vi "Store File Header.vi"(0 "∆ Trigger":dbl format="%.2f", 1 "Trigger Column":u32, 2 "Comments":string="This data's for you!\nType Command\u0011-H to get a help window for the various controls.", 4 "Offsets":dbl[](array[numeric]) format="%_6e", 6 "Scale Factors":dbl[](array[numeric]) format="%_6e", 7 "Output File Name":string, 10 "User Name":string="Conan The Scientist", 11 "File Ref Num In":refnum<file>) -> (3 "File Ref Num":refnum<file>)   [LabVIEW 2020]
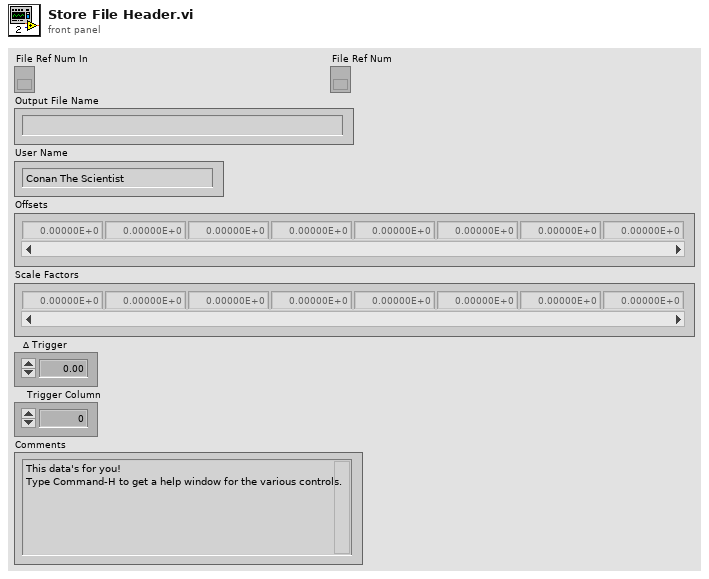
[diagram p1: front panel]
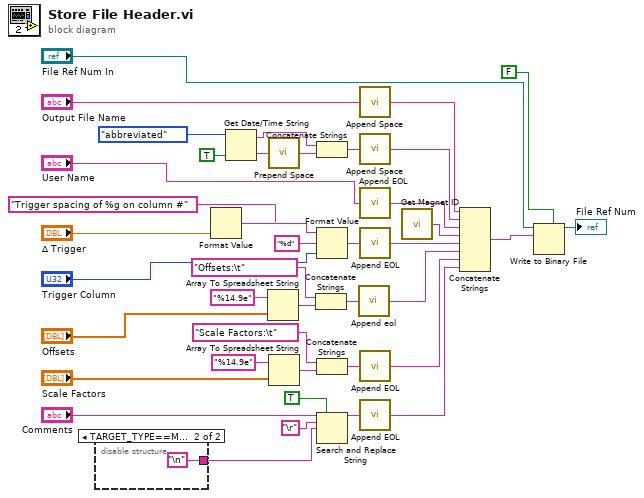
[diagram p0: block diagram]
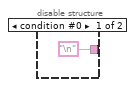
[diagram p2: hidden frame]
diagram:
  n1 = disable-structure shown="TARGET_TYPE==Mac" {
    disable-tunnel: ["\n" "\n"] -> w12
    frame condition #0 {
    }
    frame condition #1 (active) {
    }
  }
  n2 = Format Value(format string="Trigger spacing of %g on column #", value (0)="∆ Trigger") -> (output string=w31:string)  [unwired: 1 in]
  n3 = Get Date/Time String(date format (0)=enum16{"short", "long", "abbreviated"}."abbreviated", want seconds? (F)=TRUE) -> (date string=w25:string, time string=w27:string)  [unwired: 1 in]
  n4 = Array To Spreadsheet String(array="Offsets", 3:"%14.9e") -> (spreadsheet string=w4:string)  [unwired: 1 in]
  n5 = call "Prepend Space.vi"("Input String"=w27) -> ("Space + Input String"=w26:string)
  n6 = Array To Spreadsheet String(array="Scale Factors", 3:"%14.9e") -> (spreadsheet string=w38:string)  [unwired: 1 in]
  n7 = Concatenate Strings("Offsets:\t", w4) -> (w6:string)
  n8 = Concatenate Strings(w25, w26) -> (w24:string)
  n9 = Format Value(string ("")=w31, format string="%d", value (0)="Trigger Column") -> (output string=w32:string)
  n10 = Concatenate Strings("Scale Factors:\t", w38) -> (w7:string)
  n11 = Search and Replace String(replace all?=TRUE ("replace all? (F)"), input string="Comments", search string="\r", replace string=w12) -> (result string=w9:string)  [unwired: 4 in, 3 out]
  n12 = call "Append eol.vi"("INPUT STRING"=w6) -> ("OUTPUT STRING (PLUS End of Line)"=w2:string)
  n13 = call "Append Space.vi"("INPUT STRING"="Output File Name") -> ("OUTPUT STRING (PLUS [SPACE])"=w21:string)
  n14 = call "Append Space.vi"("INPUT STRING"=w24) -> ("OUTPUT STRING (PLUS [SPACE])"=w22:string)
  n15 = call "Append EOL.vi"("INPUT STRING"="User Name") -> ("OUTPUT STRING (PLUS End of Line)"=w23:string)
  n16 = call "Append EOL.vi"("INPUT STRING"=w32) -> ("OUTPUT STRING (PLUS End of Line)"=w35:string)
  n17 = call "Append EOL.vi"("INPUT STRING"=w7) -> ("OUTPUT STRING (PLUS End of Line)"=w8:string)
  n18 = call "Append EOL.vi"("INPUT STRING"=w9) -> ("OUTPUT STRING (PLUS End of Line)"=w40:string)
  n19 = call "Get Magnet ID.vi"() -> ("String"=w10:string)
  n20 = Concatenate Strings(w21, w22, w23, w10, w35, w2, w8, w40) -> (w19:string)
  n21 = Write to Binary File(file (use dialog)="File Ref Num In", data=w19, 5:FALSE ("prepend array or string size? (T)")) -> (refnum out=→"File Ref Num":refnum<file>)  [unwired: 3 in, 2 out]
